vi "Encode sfixed64.vi"(7 "Field Number":i32, 10 "sfixed64":i64, 11 "Buffer in":u8[](array[numeric]) format="%.0x") -> (3 "Buffer":u8[](array[numeric]) format="%.0x")   [LabVIEW 2020, in "LV-Proto.lvlib"]
uses:
  LV-Proto.lvlib
  Wire Type.ctl
  Wire Encode Varint I32.vi
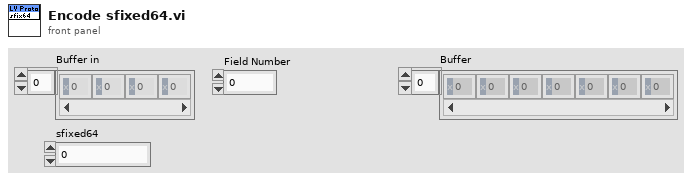
[diagram p1: front panel]
types:
  T1 = enum16{"big-endian, network order", "native, host order", "little-endian"}
  T2 = typedef "LV-Proto.lvlib/Wire Type.ctl" = enum8{"VARINT", "I64", "LEN", "SGROUP (Deprecated)", "EGROUP (Deprecated)", "I32"}
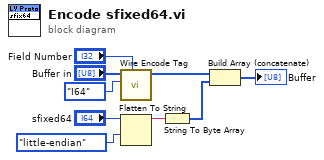
[diagram p0: block diagram]
diagram:
  n1 = call "Wire Encode Tag.vi"("Field Number"="Field Number", "Wire Type"=Wire_Type."I64", "Buffer in"="Buffer in") -> ("Buffer"=w4:u8[])  [unwired: 8 in]
  n2 = Flatten To String(anything="sfixed64", byte order (0:big-endian, network order)=T1."little-endian") -> (data string=w3:string)  [unwired: 2 in, 2 out]
  n3 = String To Byte Array(string=w3) -> (unsigned byte array=w2:u8[])
  n4 = Build Array (concatenate)(w4, w2) -> (→"Buffer":u8[])
